vi "vy_viewer.vi"(0 "picture in":picture, 2 "vy_array":T1(array[cluster]), 3 "d-distance":dbl=0.004 format="%.4f", 4 "offset":cluster{"x":i32, "y":i32}={"x"=100, "y"=100}) -> (5 "picture out":picture)   [LabVIEW 2011]
uses:
  <vilib>/Analysis/baseanly.llb/A x Vector.vi
  <vilib>/Analysis/NI_AALBase.lvlib
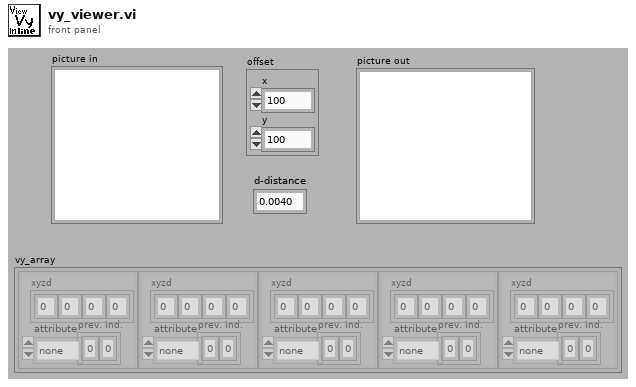
[diagram p1: front panel]
types:
  T1 = cluster{"xyzd":dbl[], "attribute":enum16{"none", "transparent", "reflective", "white", "black", "grey", "red", "yellow", "green", "blue", "pink"}, "prev. Ind.":i16[]}[]
  T2 = cluster{"xyzd":dbl[], "attribute":enum16{"none", "transparent", "reflective", "white", "black", "grey", "red", "yellow", "green", "blue", "pink"}, "prev. Ind.":i16[]}
  T3 = enum16{"transparent", "reflective", "white", "black", "red", "yellow", "green", "blue", "pink"}
  T4 = enum16{"none", "transparent", "reflective", "white", "black", "grey", "red", "yellow", "green", "blue", "pink"}
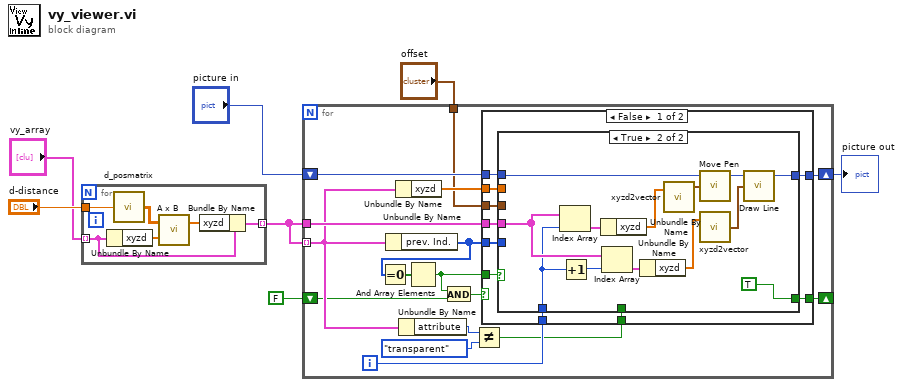
[diagram p0: block diagram]
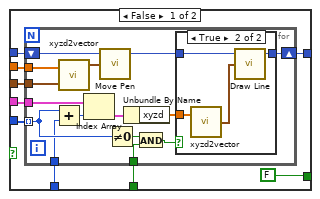
[diagram p2: hidden frame]
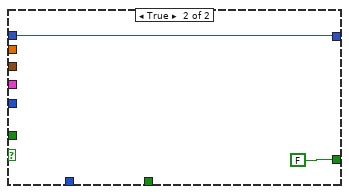
[diagram p4: hidden frame]
diagram:
  n1 = for {
    tunnel: [w11] -> w1 mode=indexing
    tunnel: "vy_array" -> [w9] mode=indexing
    tunnel: "d-distance" -> [w8]
    n2 = Unbundle By Name(w9) -> ("xyzd"=w12:dbl[])
    n3 = call "d_posmatrix.vi"("d-angle"=w8) -> ("d-matrix"=w13:dbl[][])
    n4 = call-poly <vilib>:"A x B.vi"("Vector"=w12, "A"=w13) -> ("A x Vector"=w10:dbl[])  [unwired: 1 out]
    n5 = Bundle By Name(cluster=w9, "xyzd"=w10) -> (w11:T2)
  }
  n6 = for {
    tunnel: w1 -> [w23] mode=indexing
    shift-right: [w28] -> w7
    shift-left: "picture in" -> [w29]
    tunnel: w1 -> [w26]
    tunnel: "offset" -> [w22]
    shift-right: [w17] -> _
    shift-left: FALSE -> [w14]
    i -> [w21]
    n7 = Unbundle By Name(w23) -> ("prev. Ind."=w24:i16[])
    n8 = Equal To 0?(x=w24) -> (x = 0?=w25:bool[])
    n9 = Unbundle By Name(w23) -> ("xyzd"=w27:dbl[])
    n10 = Unbundle By Name(w23) -> ("attribute"=w20:T4)
    n11 = And Array Elements(Boolean array=w25) -> (logical AND=w15:bool)
    n12 = And(x=w15, y=w14) -> (x .and. y?=w16:bool)
    n13 = Not Equal?(x=w20, y=T3."transparent" ("atribute")) -> (x != y?=w18:bool)
    n14 = case shown="False" w16 {
      tunnel: w29 -> [w39 w83]
      tunnel: [w38 w83] -> w28
      tunnel: w27 -> [w37 _]
      tunnel: w26 -> [w36 _]
      tunnel: w24 -> [w35 _]
      tunnel: w15 -> [w34 _]
      tunnel: w22 -> [w33 _]
      tunnel: w21 -> [w32 _]
      tunnel: w18 -> [w31 _]
      tunnel: [w30 FALSE] -> w17
      frame False {
        n15 = case shown="True" w34 {
          tunnel: w35 -> [w48 _]
          tunnel: w39 -> [w47 w74]
          tunnel: [w46 w73] -> w38
          tunnel: w37 -> [w45 _]
          tunnel: w36 -> [w44 w72]
          tunnel: w33 -> [w43 _]
          tunnel: w32 -> [w42 w70]
          tunnel: w31 -> [w41 _]
          tunnel: [FALSE TRUE] -> w30
          frame False {
            n16 = for {
              tunnel: w48 -> [w50] mode=indexing
              tunnel: w45 -> [w61]
              shift-right: [w62] -> w46
              shift-left: w47 -> [w63]
              tunnel: w44 -> [w60]
              tunnel: w41 -> [w53]
              tunnel: w43 -> [w52]
              tunnel: w42 -> [w49]
              n17 = Add(x=w50, y=w49) -> (x+y=w51:i32)
              n18 = call "xyzd2vector.vi"("offset"=w52, "xyzd"=w61) -> ("vector"=w57:cluster{"x":dbl, "y":dbl})
              n19 = Index Array(array=w60, index=w51) -> (element=w59:T2)
              n20 = call <vilib>:"Move Pen.vi"("new position"=w57, "picture"=w63) -> ("new picture"=w56:picture)  [unwired: 3 in]
              n21 = Not Equal To 0?(x=w50) -> (x != 0?=w54:bool)
              n22 = Unbundle By Name(w59) -> ("xyzd"=w58:dbl[])
              n23 = And(x=w54, y=w53) -> (x .and. y?=w55:bool)
              n24 = case shown="True" w55 {
                tunnel: [w64 w68] -> w62
                tunnel: w58 -> [_ w67]
                tunnel: w56 -> [w64 w66]
                frame False {
                }
                frame True {
                  n25 = call "xyzd2vector.vi"("xyzd"=w67) -> ("vector"=w65:cluster{"x":dbl, "y":dbl})  [unwired: 1 in]
                  n26 = call <vilib>:"Draw Line.vi"("picture"=w66, "end point"=w65) -> ("new picture"=w68:picture)  [unwired: 7 in]
                }
              }
            }
          }
          frame True {
            n27 = Index Array(array=w72, index=w70) -> (element=w78:T2)
            n28 = Increment(x=w70) -> (x+1=w71:i32)
            n29 = Unbundle By Name(w78) -> ("xyzd"=w77:dbl[])
            n30 = Index Array(array=w72, index=w71) -> (element=w76:T2)
            n31 = Unbundle By Name(w76) -> ("xyzd"=w75:dbl[])
            n32 = call "xyzd2vector.vi"("xyzd"=w77) -> ("vector"=w81:cluster{"x":dbl, "y":dbl})  [unwired: 1 in]
            n33 = call <vilib>:"Move Pen.vi"("new position"=w81, "picture"=w74) -> ("new picture"=w80:picture)  [unwired: 3 in]
            n34 = call "xyzd2vector.vi"("xyzd"=w75) -> ("vector"=w79:cluster{"x":dbl, "y":dbl})  [unwired: 1 in]
            n35 = call <vilib>:"Draw Line.vi"("picture"=w80, "end point"=w79) -> ("new picture"=w73:picture)  [unwired: 7 in]
          }
        }
      }
      frame True {
      }
    }
  }
  "picture out" <- w7
